vi "PH_Sequencer.PC CheckMachineStatus.vi"(0 "i ref in":refnum<vi>, 5 "error in (no error)":errorcluster) -> (14 "i ref out":refnum<vi>, 19 "error out":errorcluster)   [LabVIEW 2014, in "PH_Sequencer.lvlib"]
doc: "This VI checks the status of connected powerunits and calculates a machine status which is written to own attributes and set to the GUI."
uses:
  PH_Sequencer.lvlib
  PH_StatusHandler/PH_StatusHandler.Status.ctl
  PH_Common/PH_Common.lvlib
  PH_StatusHandler/PH_StatusHandler.lvlib
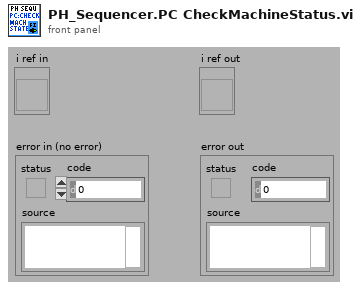
[diagram p1: front panel]
types:
  T1 = typedef "PH_StatusHandler.lvlib/PH_StatusHandler.Status.ctl" = i16
  T2 = typedef "PH_Sequencer.lvlib/PH_Sequencer.i attribute.ctl" = cluster{"GUI Refs":cluster{"Main Off":refnum<vi>, "Fire":refnum<vi>, "Status":refnum<vi>, "Ready":refnum<vi>, "Waiting Time":refnum<vi>, "Timeout":refnum<vi>, "PPMA Ready":refnum<vi>, "Sequencer SM State":refnum<vi>, "PPPA Ready":refnum<vi>, "Calorimeter":refnum<vi>, "Beamline Ready":refnum<vi>, "Clear Beamline":refnum<vi>, "Linkage PPMA Rods":refnum<vi>, "Linkage Current PA":refnum<vi>, "Linkage Current MA":refnum<vi>, "Timing Ready":refnum<vi>, "State Timing":refnum<vi>, "Force Timing":refnum<vi>, "PSDB Shot Comment":refnum<vi>, "State PA Backreflection":refnum<vi>, "Beamline Z6 Ready":refnum<vi>, "Clear Z6 Beamline":refnum<vi>, "Sequence length":refnum<vi>, "Timing Mode":refnum<vi>, "Slow Trigger Settings":refnum<vi>, "Experiment Description":refnum<vi>, "State PSDB":refnum<vi>, "PSDB Ready":refnum<vi>, "Set PSDB Settings":refnum<vi>, "Get PSDB Info":refnum<vi>, "Take Snapshot":refnum<vi>, "Shottype":refnum<vi>, "Experiment":refnum<vi>, "Phase Frontends":refnum<vi>, "PP 45mm PILC in use":refnum<vi>}, "Status Info":cluster{"Machine Status":T1, "WaitingTime":i32, "Timeout":bool}, "Readyness":cluster{"Ready to shot":bool, "PPMA Ready":bool, "PPPA Ready":bool, "BL Ready":bool, "Timing Ready":bool, "BL Z6 Ready":bool, "PSDBReady":bool}, "Instancenames":cluster{"PPMA Rods":string, "PP Current Meas":string, "PH Beamline Chief":string, "PA Backrefl Meas":string, "Z6 Beamline Chief":string}, "Data to read":bool, "Calorimeter":cluster{"Instancename":string, "On":bool, "linked":bool}, "Linkage":cluster{"PPMA Rods":bool, "PP Current Meas":bool, "PHELIX Beamline Chief":bool, "PA Backrefl Meas":bool, "Z6 Beamline Chief":bool}, "Timing":cluster{"Instance":string, "linked":bool, "Status":T1, "Timing Mode":T3, "Slow Trigger Settings":T4, "Info available":cluster{"ext SlowTrigger":bool, "T2":bool, "Mode":bool, "Delay Slow Trigger":bool, "Phase FEs":bool}, "FE Phase":T5}, "Service ID R2S":i32, "PSDB":cluster{"Controller Instance":string, "Controller Status":T1, "Controller linked":bool, "Settings acknowledged":bool, "Current Experiment ID":i16, "Current Shot Type":i16, "Current Comment":string, "Remember Settings":bool, "Write 2 early":bool}, "PSDB Data":cluster{"Main Off?":bool, "Sequence Length":dbl, "Sequence startet":timestamp}, "6P 4Q Positions":cluster{"Instancename":string, "linked":bool, "Position":T6}[], "PUs":T7[]}
  T3 = typedef "PH_Timing.lvlib/PH_Timing.Timing Mode.ctl" = cluster{"T2":i16, "Modeselector":enum32{"10 Hz", "0.5 Hz", "Shot"}}
  T4 = typedef "PH_Timing.lvlib/PH_Timing.Slow Trigger Settings.ctl" = cluster{"Delay":dbl, "externally triggered?":bool}
  T5 = typedef "PH_Timing.lvlib/PH_Timing.Phase FEs.ctl" = cluster{"Phase":dbl}
  T6 = typedef "PH_4_Pos_Selector.lvlib/PH_4_Pos_Selector.Position Selector.ctl" = u16
  T7 = typedef "PH_Sequencer.lvlib/PH_Sequencer.Head.ctl" = cluster{"PowerUnit":T8, "GUI Ref":refnum<vi>, "Information":T9, "linked?":bool, "GUI Ref Current Voltage":refnum<vi>}
  T8 = typedef "PH_PP_Common.lvlib/PH_PP_Common.PUs.ctl" = enum16{"no Info", "PA-19mm-1", "PA-19mm-2", "PA-45mm-PILC", "PA-45mm-MAIN", "MA-PU-1", "MA-PU-2", "MA-PU-3", "MA-PU-4", "MA-PU-5", "MA-PU-6", "MA-FR", "MA-PILC", "PA-45mm-DP"}
  T9 = typedef "PH_Sequencer.lvlib/PH_Sequencer.PU Information.ctl" = cluster{"State":T1, "Waiting Time [s]":dbl, "PU State SM":T10, "PU Timeout SM":T10}
  T10 = typedef "PH_PowerUnit_BaseClass.lvlib/PH_PowerUnit_BaseClass.SM States.ctl" = enum16{".", "Stand by", "Switch PU on", "Configure", "Set Default Voltage", "Set STANDBY", "Set READY", "Wait for Shot Cmd", "Open Dump Rods", "Open Ross Relais", "Close Ross Relais", "Switch PSU on", "Switch PSU off", "Charge", "Switch GD Channel on", "Close Dump Rods", "Rods-TO", "RR-TO", "PSU-TO", "Trigger-TO"}
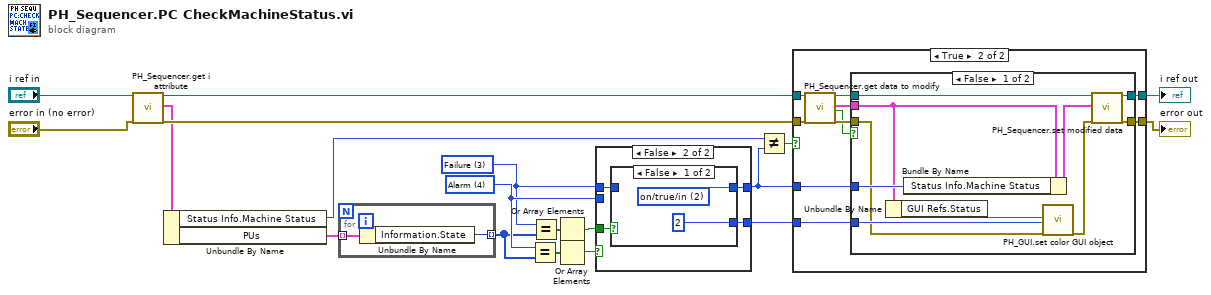
[diagram p0: block diagram]
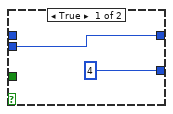
[diagram p4: hidden frame]
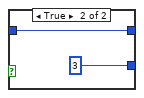
[diagram p5: hidden frame]
diagram:
  w6 = T1 3 items=["no info", "off/false/out", "on/true/in", "Failure", "Alarm", "Status 1", "Status 2", "Status 3"] ("PU 19mm - 1.State")
  w7 = T1 4 items=["no info", "off/false/out", "on/true/in", "Failure", "Alarm", "Status 1", "Status 2", "Status 3"] ("PU 19mm - 1.State")
  n1 = call "PH_Sequencer.get i attribute.vi"("i ref in"="i ref in", "error in (no error)"="error in (no error)") -> ("i ref out"=w18:refnum<vi>, "i attribute"=w15:T2, "error out"=w16:errorcluster)  [unwired: 15 in]
  n2 = Unbundle By Name(w15) -> ("Status Info.Machine Status"=w4:T1, "PUs"=w1:T7[])
  n3 = for {
    tunnel: w1 -> [w21] mode=indexing
    tunnel: [w20] -> w5 mode=indexing
    n4 = Unbundle By Name(w21) -> ("Information.State"=w20:T1)
  }
  n5 = Equal?(x=w7, y=w5) -> (x = y?=w12:bool[])
  n6 = Equal?(x=w6, y=w5) -> (x = y?=w10:bool[])
  n7 = Or Array Elements(Boolean array=w10) -> (logical OR=w9:bool)
  n8 = Or Array Elements(Boolean array=w12) -> (logical OR=w11:bool)
  n9 = case shown="False" w11 {
    tunnel: w9 -> [_ w27]
    tunnel: [w23 w26] -> w3
    tunnel: w6 -> [_ w25]
    tunnel: w7 -> [w23 _]
    tunnel: [4 w24] -> w8
    frame True {
    }
    frame False {
      n10 = case shown="False" w27 {
        tunnel: [w28 w31] -> w26
        tunnel: w25 -> [_ w31]
        tunnel: [2 3] -> w24
        frame False {
          w28 = T1 2 items=["no info", "off/false/out", "on/true/in", "Failure", "Alarm", "Status 1", "Status 2", "Status 3"] ("PU 19mm - 1.State")
        }
        frame True {
        }
      }
    }
  }
  n11 = Not Equal?(x=w4, y=w3) -> (x != y?=w2:bool)
  n12 = case shown="True" w2 {
    tunnel: [w33 w43] -> w19
    tunnel: w18 -> [w33 w42]
    tunnel: [w32 w41] -> w17
    tunnel: w16 -> [w32 w40]
    tunnel: w8 -> [_ w39]
    tunnel: w3 -> [_ w34]
    frame False {
    }
    frame True {
      n13 = call "PH_Sequencer.get data to modify.vi"("i ref in"=w42, "error in (no error)"=w40) -> ("i ref out"=w37:refnum<vi>, "i attribute"=w36:T2, "timed out"=w35:bool, "error out"=w38:errorcluster)  [unwired: 14 in]
      n14 = case shown="False" w35 {
        tunnel: [w53 w55] -> w43
        tunnel: [w52 w54] -> w41
        tunnel: w34 -> [w49 _]
        tunnel: w39 -> [w48 _]
        tunnel: w38 -> [w47 w54]
        tunnel: w37 -> [w46 w55]
        tunnel: w36 -> [w45 _]
        frame False {
          n15 = Unbundle By Name(w45) -> ("GUI Refs.Status"=w44:refnum<vi>)
          n16 = Bundle By Name(cluster=w45, "Status Info.Machine Status"=w49) -> (w50:T2)
          n17 = call "PH_GUI.set color GUI object.vi"("GUI object Ref"=w44, "State"=w48, "error in (no error)"=w47) -> ("error out"=w51:errorcluster)  [unwired: 16 in]
          n18 = call "PH_Sequencer.set modified data.vi"("i ref in"=w46, "i attribute"=w50, "error in (no error)"=w51) -> ("i ref out"=w53:refnum<vi>, "error out"=w52:errorcluster)  [unwired: 15 in]
        }
        frame True {
        }
      }
    }
  }
  "i ref out" <- w19
  "error out" <- w17
